vi "Generate Linear Accel Segment.vi"(6 "Index":i32, 7 "Initial Acceleration":dbl format="%#_13g", 9 "Linear Info":T2, 11 "Speeds":T1={"maxV (fps)"=20.0, "Accel Limit (fps^2)"=20.0, "Initial V (fps)"=0.0, "Sample Period (s)"=0.02, "Jerk Limit (fps^3)"=0.0, "Front Distances"={"distance (ft)"=0.0, "baseline (ft)"=0.0, "high (ft)"=0.0}, "Back Distances"={"distance (ft)"=0.0, "baseline (ft)"=0.0, "high (ft)"=0.0}}) -> (0 "Valid":bool, 1 "Final Position":cluster{dbl, dbl, dbl}, 2 "Trajectory Segment":T3, 3 "Speeds Out":T1={"maxV (fps)"=0.0, "Accel Limit (fps^2)"=0.0, "Initial V (fps)"=0.0, "Sample Period (s)"=0.02, "Jerk Limit (fps^3)"=0.0, "Front Distances"={"distance (ft)"=0.0, "baseline (ft)"=0.0, "high (ft)"=0.0}, "Back Distances"={"distance (ft)"=0.0, "baseline (ft)"=0.0, "high (ft)"=0.0}}, 5 "Final Acceleration":dbl)   [LabVIEW 2018]
panel:
  out "Waveform Graph":dbl[][](graph)
  out "XY Graph":cluster{dbl, dbl}[](graph)
  out "Segment Time (s)":dbl
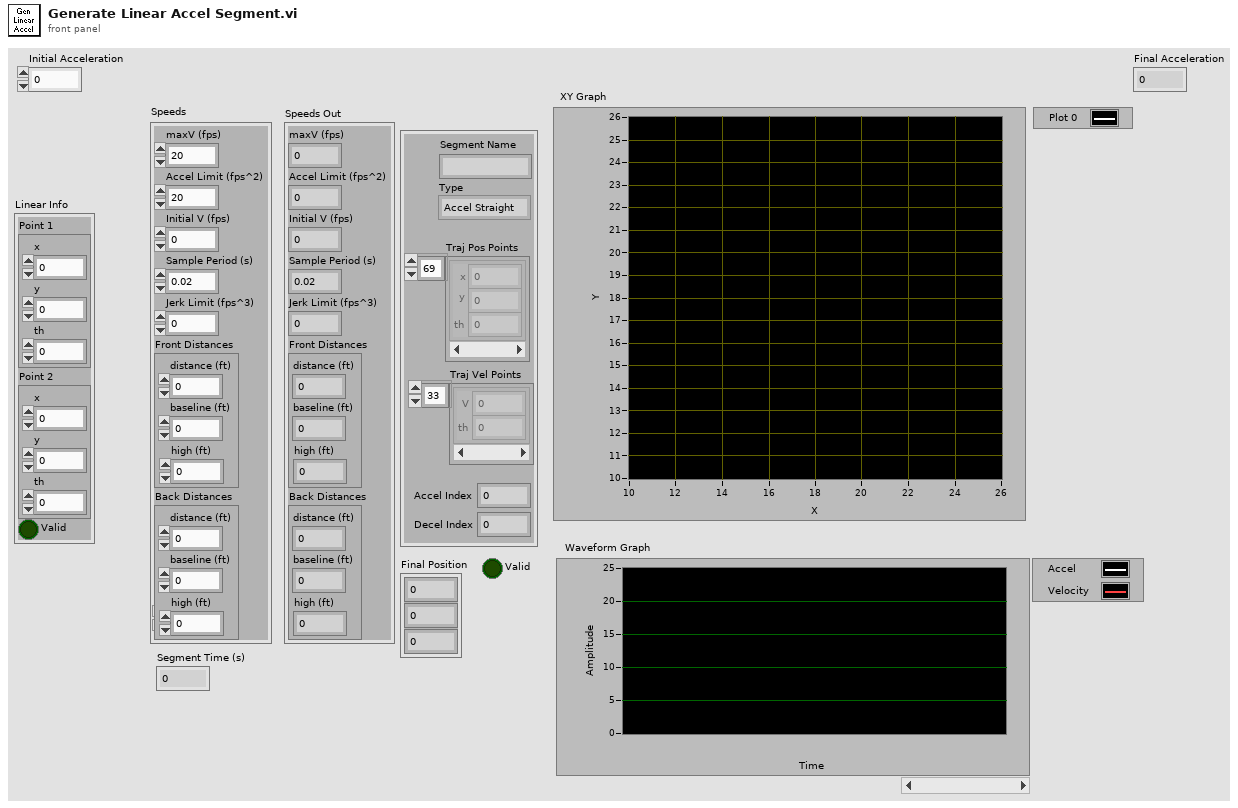
[diagram p1: front panel]
types:
  T1 = cluster{"maxV (fps)":dbl, "Accel Limit (fps^2)":dbl, "Initial V (fps)":dbl, "Sample Period (s)":dbl, "Jerk Limit (fps^3)":dbl, "Front Distances":cluster{"distance (ft)":dbl, "baseline (ft)":dbl, "high (ft)":dbl}, "Back Distances":cluster{"distance (ft)":dbl, "baseline (ft)":dbl, "high (ft)":dbl}}
  T2 = cluster{"Point 1":cluster{"x":dbl, "y":dbl, "th":dbl}, "Point 2":cluster{"x":dbl, "y":dbl, "th":dbl}, "Valid":bool}
  T3 = cluster{"Segment Name":string, "Type":enum16{"Accel Straight", "Const Straight", "Blend", "Circle"}, "Traj Pos Points":cluster{"x":dbl, "y":dbl, "th":dbl}[], "Traj Vel Points":cluster{"V":dbl, "th":dbl}[], "Accel Index":i32, "Decel Index":i32}
  T4 = enum16{"Accel Straight", "Const Straight", "Blend", "Circle"}
  T5 = cluster{"distance (ft)":dbl, "baseline (ft)":dbl, "high (ft)":dbl}
  T6 = cluster{"Initial Acceleration":dbl, "Initial V (fps)":dbl}
  T7 = cluster{string, "Type":enum16{"Accel Straight", "Const Straight", "Blend", "Circle"}, cluster{dbl, dbl, dbl}[], cluster{"velocity":dbl, dbl}[], "Accel Index":i32, "Decel Index":i32}
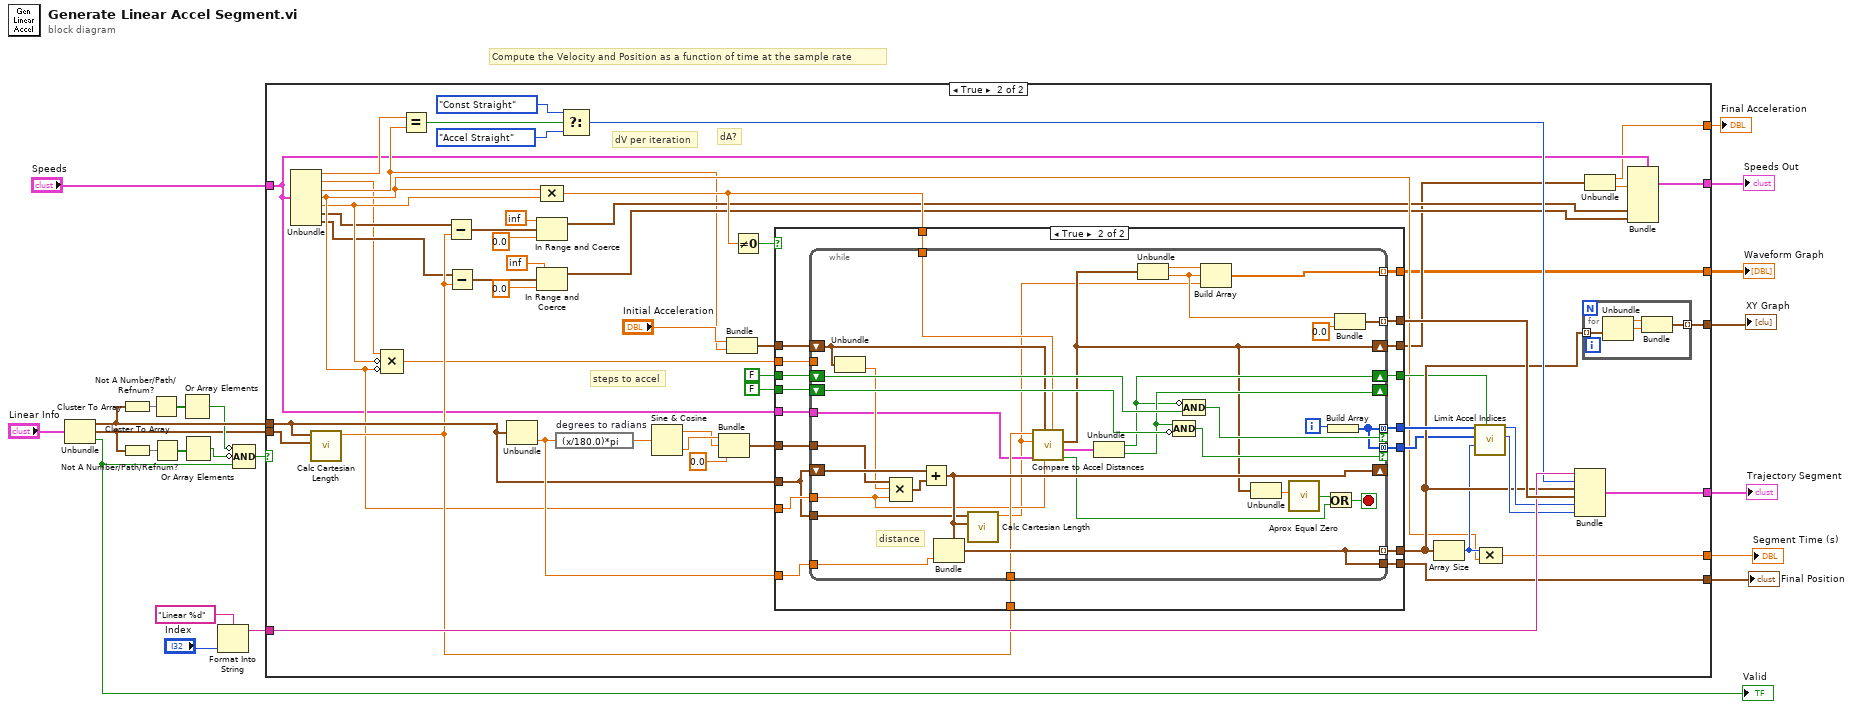
[diagram p0: block diagram]
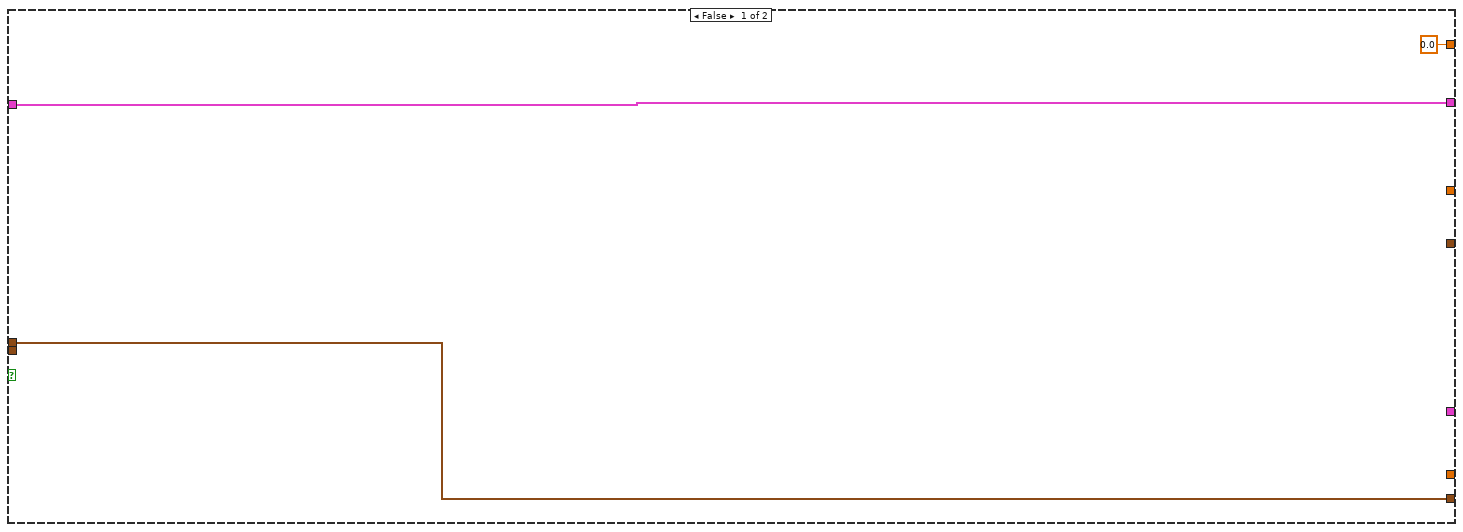
[diagram p2: hidden frame]
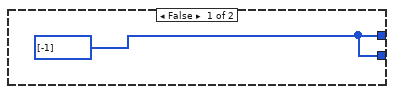
[diagram p3: hidden frame]
diagram:
  # "Compute the Velocity and Position as a function of time at the sample rate"
  n1 = Unbundle("Linear Info") -> ("Point 1"=w10:cluster{"x":dbl, "y":dbl, "th":dbl}, "Point 2"=w5:cluster{"x":dbl, "y":dbl, "th":dbl}, "Valid"=w11:bool)
  "Valid" <- w11
  n2 = Cluster To Array(cluster=w10) -> (array=w9:dbl[])
  n3 = Cluster To Array(cluster=w5) -> (array=w6:dbl[])
  n4 = Not A Number/Path/Refnum?(number/path/refnum=w9) -> (NaN/Path/Refnum?=w8:bool[])
  n5 = Not A Number/Path/Refnum?(number/path/refnum=w6) -> (NaN/Path/Refnum?=w4:bool[])
  n6 = Or Array Elements(Boolean array=w8) -> (logical OR=w7:bool)
  n7 = Or Array Elements(Boolean array=w4) -> (logical OR=w3:bool)
  n8 = Format Into String(format string="Linear %d", "Index") -> (resulting string=w14:string)  [unwired: 2 in, 1 out]
  n9 = Compound Arithmetic op=AND(invert w7, invert w3, w11) -> (w12:bool)
  n10 = case shown="True" w12 {
    tunnel: [_ w79] -> w22
    tunnel: w14 -> [_ w73]
    tunnel: [_ w69] -> w21
    tunnel: [w24 w68] -> w20
    tunnel: [_ w65] -> w19
    tunnel: "Speeds" -> [w25 w27]
    tunnel: [w25 w64] -> w17
    tunnel: w10 -> [w24 w58]
    tunnel: w5 -> [_ w61]
    tunnel: [_ w28] -> w2
    tunnel: [0.0 w26] -> w1
    frame False {
    }
    frame True {
      # "dA?"
      # "steps to accel"
      # "dV per iteration"
      n11 = Unbundle(w27) -> ("maxV (fps)"=w63:dbl, "Accel Limit (fps^2)"=w29:dbl, "Initial V (fps)"=w33:dbl, "Sample Period (s)"=w41:dbl, "Jerk Limit (fps^3)"=w39:dbl, "Front Distances"=w38:T5, "Back Distances"=w35:T5)
      n12 = call "Calc Cartesian Length.vi"("Point 2"=w61, "Point 1"=w58) -> ("Length (f)"=w49:dbl)  [unwired: 8 in, 1 out]
      n13 = Compound Arithmetic op=MULTIPLY(w29, invert w39, invert w41) -> (w42:dbl)
      n14 = Equal?(x=w63, y=w33) -> (x = y?=w62:bool)
      n15 = Subtract(x=w38, y=w49) -> (x-y=w54:T5)
      n16 = Subtract(x=w35, y=w49) -> (x-y=w48:T5)
      n17 = Unbundle(w58) -> ("th"=w67:dbl)  [unwired: 2 out]
      n18 = In Range and Coerce(upper limit=inf, x=w54, lower limit=0.0) -> (coerced(x)=w37:T5)  [unwired: 1 out]
      n19 = In Range and Coerce(upper limit=inf, x=w48, lower limit=0.0) -> (coerced(x)=w36:T5)  [unwired: 1 out]
      n20 = Compound Arithmetic op=MULTIPLY(w41, w39) -> (w60:dbl)
      n21 = expression code="(x/180.0)*pi" "degrees to radians"(w67) -> (w66:dbl)
      n22 = Select(t=T4."Const Straight" ("Type"), s=w62, f=T4."Accel Straight" ("Type")) -> (s? t:f=w70:T4)
      n23 = Sine & Cosine(0:w66) -> (1:w74:dbl, 2:w75:dbl)
      n24 = Bundle(w75, w74, 0.0) -> (w77:cluster{dbl, dbl, dbl})  [unwired: 1 in]
      n25 = Bundle("Initial Acceleration"="Initial Acceleration", "Initial V (fps)"=w33) -> (w32:T6)  [unwired: 1 in]
      n26 = Not Equal To 0?(x=w60) -> (x != 0?=w59:bool)
      n27 = case shown="True" w59 {
        tunnel: [_ w103] -> w78
        tunnel: w77 -> [_ w102]
        tunnel: [_ w101] -> w68
        tunnel: w67 -> [_ w100]
        tunnel: [_ w99] -> w46
        tunnel: [_ w98] -> w31
        tunnel: w60 -> [_ w97]
        tunnel: w41 -> [_ w96]
        tunnel: w58 -> [_ w95]
        tunnel: w49 -> [_ w94]
        tunnel: FALSE -> [_ w93]
        tunnel: [w84 w92] -> w52
        tunnel: w27 -> [_ w91]
        tunnel: FALSE -> [_ w90]
        tunnel: [w84 w89] -> w45
        tunnel: [_ w88] -> w43
        tunnel: w42 -> [_ w87]
        tunnel: w32 -> [_ w86]
        tunnel: [_ w85] -> w28
        frame False {
          w84 = i32[] [-1]
        }
        frame True {
          n28 = while {
            tunnel: [w128] -> w99 mode=indexing
            tunnel: w97 -> [w112]
            shift-right: [w105] -> w98
            shift-left: w86 -> [w116]
            tunnel: [w134] -> w103 mode=indexing
            tunnel: w96 -> [w109]
            tunnel: w102 -> [w132]
            tunnel: w100 -> [w135]
            tunnel: [w128] -> w101
            tunnel: w94 -> [w126]
            shift-right: [w130] -> _
            shift-left: w95 -> [w133]
            tunnel: w95 -> [w129]
            shift-right: [w111] -> w88
            shift-left: w93 -> [w125]
            tunnel: [w122] -> w92 mode=concatenating if=w124
            tunnel: w91 -> [w108]
            shift-right: [w114] -> _
            shift-left: w90 -> [w123]
            tunnel: [w122] -> w89 mode=concatenating if=w121
            tunnel: w87 -> [_]
            tunnel: [w110] -> w85 mode=indexing
            i -> [w127]
            stop <- w119 stop-if-true
            # "distance"
            n29 = Unbundle(w116) -> ("Initial V (fps)"=w117:dbl)  [unwired: 1 out]
            n30 = Compound Arithmetic op=MULTIPLY(w132, w117, w109) -> (w131:cluster{dbl, dbl, dbl})
            n31 = Add(x=w133, y=w131) -> (x+y=w130:cluster{dbl, dbl, dbl})
            n32 = Bundle(cluster=w130, w135) -> (w128:cluster{dbl, dbl, dbl})  [unwired: 2 in]
            n33 = call "Calc Cartesian Length.vi"("Point 2"=w130, "Point 1"=w129) -> ("Length (f)"=w104:dbl)  [unwired: 8 in, 1 out]
            n34 = call "Compare to Accel Distances.vi"("dA"=w112, "Sample Period (s)"=w109, "Values"=w116, "Speeds"=w108, "Current  Length"=w104, "Total Segment Length"=w126) -> ("End Loop"=w120:bool, "Ends"=w115:cluster{"Accel End":bool, "Decel End":bool}, "Values out"=w105:cluster{"accel":dbl, "velocity":dbl})  [unwired: 2 in, 1 out]
            n35 = Unbundle(w115) -> ("Accel End"=w111:bool, "Decel End"=w114:bool)
            n36 = Unbundle(w105) -> ("accel"=w106:dbl, "velocity"=w107:dbl)
            n37 = Compound Arithmetic op=AND(w114, invert w123) -> (w121:bool)
            n38 = Compound Arithmetic op=AND(invert w111, w125) -> (w124:bool)
            n39 = Build Array(w106, w107, w104) -> (w110:dbl[])
            n40 = Unbundle(w105) -> ("velocity"=w113:dbl)  [unwired: 1 out]
            n41 = call "Aprox Equal Zero.vi"("maxV (fps)"=w113) -> ("Boolean"=w118:bool)  [unwired: 10 in]
            n42 = Or(x=w118, y=w120) -> (x .or. y?=w119:bool)
            n43 = Build Array(w127) -> (w122:i32[])
            n44 = Bundle("velocity"=w107, 0.0) -> (w134:cluster{"velocity":dbl, dbl})  [unwired: 1 in]
          }
        }
      }
      n45 = Array Size(array=w46) -> (size(s)=w44:i32)
      n46 = call "Limit Accel Indices.vi"("Last Accel"=w43, "Size"=w44, "Decel"=w45, "Accel"=w52) -> ("Decel Index"=w51:i32, "Accel Index"=w53:i32)  [unwired: 6 in]
      n47 = Compound Arithmetic op=MULTIPLY(w44, w41) -> (w69:dbl)
      n48 = Bundle(w73, "Type"=w70, w46, w78, "Accel Index"=w53, "Decel Index"=w51) -> (w79:T7)  [unwired: 1 in]
      n49 = for {
        tunnel: w46 -> [w83] mode=indexing
        tunnel: [w80] -> w65 mode=indexing
        n50 = Unbundle(w83) -> (w82:dbl, w81:dbl)  [unwired: 1 out]
        n51 = Bundle(w82, w81) -> (w80:cluster{dbl, dbl})  [unwired: 1 in]
      }
      n52 = Unbundle(w31) -> ("Initial Acceleration"=w26:dbl, "Initial V (fps)"=w30:dbl)
      n53 = Bundle(cluster=w27, "Initial V (fps)"=w30, "Front Distances"=w37, "Back Distances"=w36) -> (w64:T1)  [unwired: 4 in]
    }
  }
  "Trajectory Segment" <- w22
  "Segment Time (s)" <- w21
  "Final Position" <- w20
  "XY Graph" <- w19
  "Speeds Out" <- w17
  "Waveform Graph" <- w2
  "Final Acceleration" <- w1
